vi "CreateTextFile.vi"(11 "Input File Path":path) -> ()   [LabVIEW 2023, in "FileUtilities.lvlib"]
uses:
  FileUtilities.lvlib
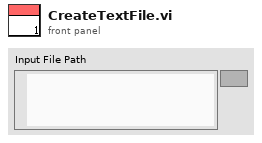
[diagram p1: front panel]
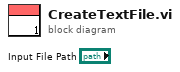
[diagram p0: block diagram]
diagram:
